vi "Zeitstempel in String Umwandeln.vi"() -> (0 "Zeitstempel":string, 2 "Zeitstempel mit Kommastellen":string)   [LabVIEW 2020, in "allgemeine Sub-VIs.lvlib"]
uses:
  allgemeine Sub-VIs.lvlib
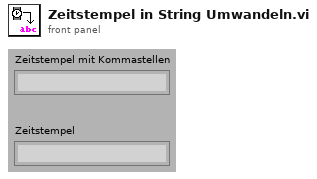
[diagram p1: front panel]
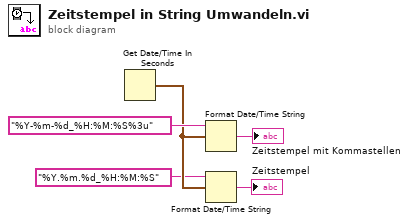
[diagram p0: block diagram]
diagram:
  n1 = Get Date/Time In Seconds() -> (seconds since 1Jan1904=w3:timestamp)
  n2 = Format Date/Time String(time format string (%c)="%Y-%m-%d_%H:%M:%S%3u" ("Zeitformatierungs-String (%c)"), seconds (now)=w3) -> (date/time string=→"Zeitstempel mit Kommastellen":string)  [unwired: 1 in]
  n3 = Format Date/Time String(time format string (%c)="%Y.%m.%d_%H:%M:%S" ("Zeitformatierungs-String (%c)"), seconds (now)=w3) -> (date/time string=→"Zeitstempel":string)  [unwired: 1 in]
